vi "Get Default Parent Message Class Path.vi"(8 "error in (no error)":errorcluster, 11 "Message Scripter":refnum<class "Message Scripter.lvclass">) -> (0 "error out":errorcluster, 2 "Path String":path)   [LabVIEW 2020, in "Message Maker.lvlib" / "Message Scripter.lvclass"]
uses:
  Message Scripter.lvclass
  Message Maker.lvlib
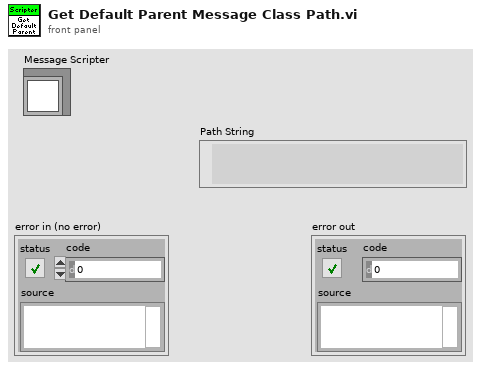
[diagram p1: front panel]
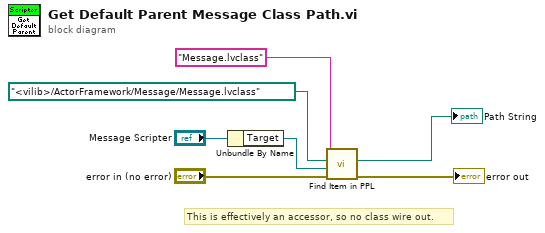
[diagram p0: block diagram]
diagram:
  # "This is effectively an accessor, so no class wire out."
  n1 = Unbundle By Name("Message Scripter") -> ("Target"=w3:refnum<vi>)
  n2 = call "Find Item in PPL.vi"("error in (no error)"="error in (no error)", "Target"=w3, "default path"=path "<vilib>/ActorFramework/Message/Message.lvclass" ("Path"), "qualified name"="Message.lvclass" ("key")) -> ("error out"=→"error out":errorcluster, "item path out"=→"Path String":path)  [unwired: 5 in, 1 out]
